vi "Generate Async Msg Event.vi"(7 "AdHoc Msg (\"\")":string, 8 "error in (no error)":errorcluster, 9 "vData":variant, 10 "AsyncMsg":T1, 11 "DbgTimers in":refnum<class "DbgTimers.lvclass">) -> (0 "error out":errorcluster, 3 "DbgTimers out":refnum<class "DbgTimers.lvclass">)   [LabVIEW 2017, in "DbgTimers.lvclass"]
doc: "Developed by Kevin Thompson\nkevin@thompsonengineering.net\n\nCopyright 2018-2020\nThompson Engineering, LLC"
uses:
  DbgTimers.lvclass
  DataTypes/AsynMsg_DbgTimers--enum.ctl
  Ichor_Common/DataTypes/TD Async CmdMsg EventData--cluster.ctl
  DbgTimers.lvclass/DbgTimers.ctl
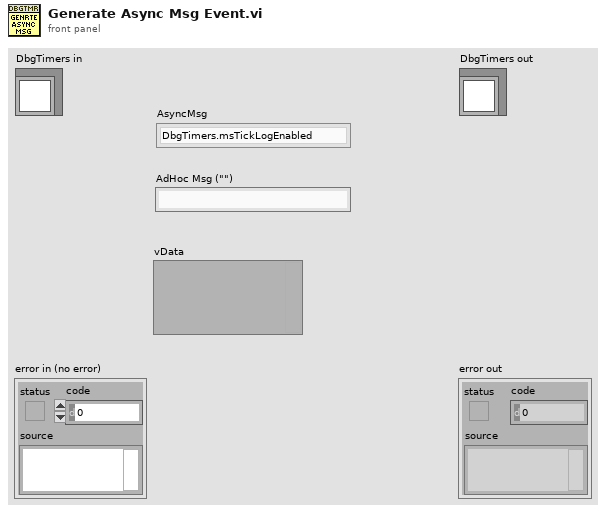
[diagram p1: front panel]
types:
  T1 = typedef "DbgTimers.lvclass/AsynMsg_DbgTimers--enum.ctl" = enum16{"DbgTimers.msTickLogEnabled"}
  T2 = typedef "TD Async CmdMsg EventData--cluster.ctl" = cluster{"Time Stamp":timestamp, "CmdMsg":string, "vData":variant}
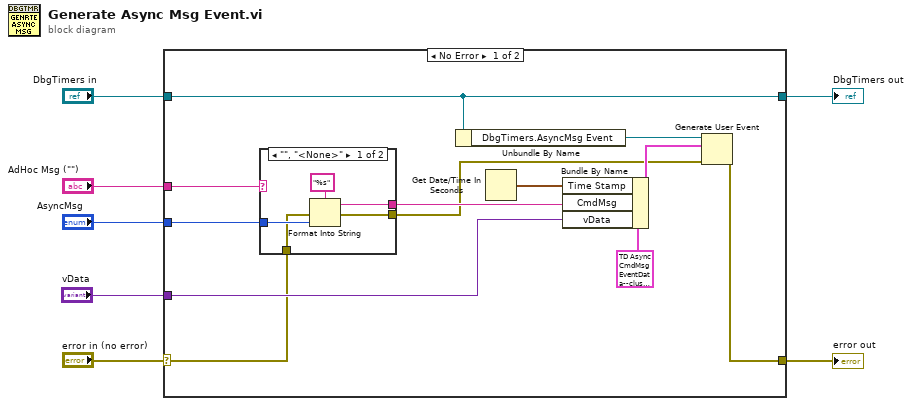
[diagram p0: block diagram]
diagram:
  n1 = case shown="No Error" "error in (no error)" {
    selector: "error in (no error)" -> [w11 w28]
    tunnel: [w18 w28] -> w2
    tunnel: [w12 w27] -> w6
    tunnel: "DbgTimers in" -> [w12 w27]
    tunnel: "AsyncMsg" -> [w9 _]
    tunnel: "vData" -> [w13 _]
    tunnel: "AdHoc Msg (\"\")" -> [w8 _]
    frame No Error {
      n2 = case shown="\"\", \"<None>\"" w8 {
        selector: w8 -> [_ w25]
        tunnel: w9 -> [w23 _]
        tunnel: [w22 w25] -> w14
        tunnel: w11 -> [w21 w26]
        tunnel: [w20 w26] -> w10
        frame "", "<None>" {
          n3 = Format Into String(format string="%s", error in=w21, w23) -> (resulting string=w22:string, error out=w20:errorcluster)  [unwired: 1 in]
        }
        frame Default {
        }
      }
      n4 = Unbundle By Name(w12) -> ("DbgTimers.AsyncMsg Event"=w19:refnum<user-event>)
      n5 = Get Date/Time In Seconds() -> (seconds since 1Jan1904=w15:timestamp)
      n6 = Bundle By Name(cluster=T2 {"Time Stamp"=timestamp(0 s since 1904-01-01), "CmdMsg"="", "vData"=variant} ("Async EvData"), "Time Stamp"=w15, "CmdMsg"=w14, "vData"=w13) -> (w17:T2)
      n7 = Generate User Event(user event=w19, event data cluster=w17, error in=w10) -> (error out=w18:errorcluster)  [unwired: 1 in, 1 out]
    }
    frame Error {
    }
  }
  "error out" <- w2
  "DbgTimers out" <- w6
